vi "MBus Data Sort.vi"(3 "Error In":errorcluster, 4 "Raw Input Data":bool[](array[boolean]), 5 "Modbus master in":refnum<class "Modbus Master.lvclass">) -> (0 "Error Out":errorcluster, 1 "Cmd Value":bool[](array[boolean]), 2 "Modbus master out":refnum<class "Modbus Master.lvclass">)   [LabVIEW 2018]
uses:
  <vilib>/NI/Modbus Library/API/master/Modbus Master.lvclass
  CTL/FGV - R-W.ctl
panel:
  out "Supply 1 Voltage":u32
  out "Supply 2 Voltage":u32
  out "Remainder Data":bool[](array[boolean])
  out "Flash FB":bool[](array[boolean])
  out "Fault FB":bool[](array[boolean])
  out "Supply 2 Value":bool[](array[boolean])
  out "Supply 1 Value":bool[](array[boolean])
  out "System FB":bool[](array[boolean])
  out "Spares":bool[](array[boolean])
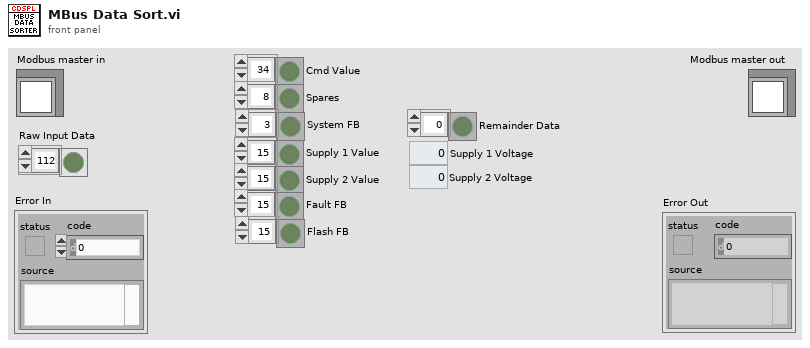
[diagram p1: front panel]
types:
  T1 = typedef "FGV - R-W.ctl" = enum16{"W", "R"}
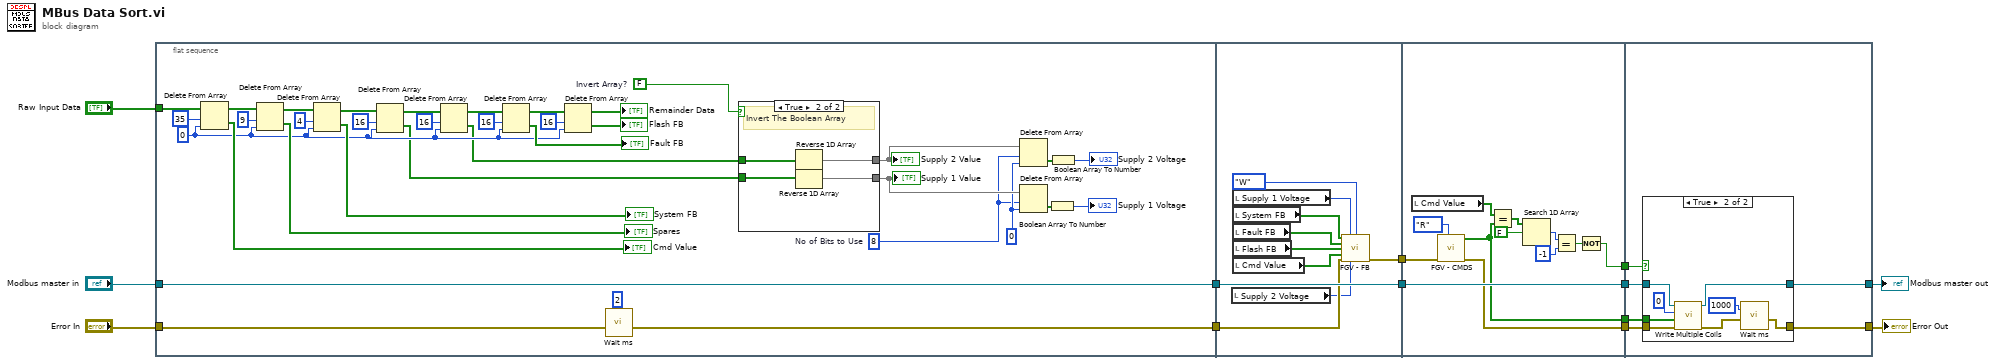
[diagram p0: block diagram]
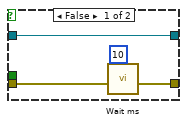
[diagram p3: hidden frame]
diagram:
  n1 = flat-sequence {
    tunnel: "Raw Input Data" -> [w49]
    tunnel: "Error In" -> [w16]
    tunnel: [w15] -> w10
    tunnel: "Modbus master in" -> [w14]
    tunnel: [w14] -> w8
    tunnel: w10 -> [w64]
    tunnel: w8 -> [w65]
    tunnel: [w63] -> w6
    tunnel: [w65] -> w5
    tunnel: w6 -> [w66]
    tunnel: w5 -> [w77]
    tunnel: [w75] -> w4
    tunnel: [w77] -> w3
    tunnel: [w68] -> w2
    tunnel: [w67] -> w1
    tunnel: [w80] -> w7
    tunnel: [w79] -> w11
    tunnel: w4 -> [w83]
    tunnel: w3 -> [w81]
    tunnel: w2 -> [w82]
    tunnel: w1 -> [w78]
    frame #0 {
      w22 = 8  # No of Bits to Use
      w23 = 0 ("index")
      w28 = FALSE  # Invert Array?
      w31 = 0 ("index")
      n2 = Delete From Array(array=w49, length=35, index=w31) -> (deleted portion=→"Cmd Value":bool[], array with subset deleted=w46:bool[])
      n3 = Delete From Array(array=w46, length=9, index=w31) -> (deleted portion=→"Spares":bool[], array with subset deleted=w43:bool[])
      n4 = Delete From Array(array=w43, length=4, index=w31) -> (deleted portion=→"System FB":bool[], array with subset deleted=w39:bool[])
      n5 = Delete From Array(array=w39, length=16, index=w31) -> (deleted portion=w26:bool[], array with subset deleted=w37:bool[])
      n6 = Delete From Array(array=w37, length=16, index=w31) -> (deleted portion=w27:bool[], array with subset deleted=w35:bool[])
      n7 = Delete From Array(array=w35, length=16, index=w31) -> (deleted portion=→"Fault FB":bool[], array with subset deleted=w33:bool[])
      n8 = Delete From Array(array=w33, length=16, index=w31) -> (deleted portion=→"Flash FB":bool[], array with subset deleted=→"Remainder Data":bool[])
      n9 = call "Wait ms.vi"("milliseconds to wait"=u32 2, "error in (no error)"=w16) -> ("error out"=w15:errorcluster)  [unwired: 9 in]
      n10 = case shown="True" w28 {
        tunnel: w27 -> [w51 w55]
        tunnel: [w51 w54] -> w25
        tunnel: w26 -> [w50 w53]
        tunnel: [w50 w52] -> w24
        frame False {
          # "Use Array as it is"
        }
        frame True {
          # "Invert The Boolean Array"
          n11 = Reverse 1D Array(array=w55) -> (reversed array=w54:bool[])
          n12 = Reverse 1D Array(array=w53) -> (reversed array=w52:bool[])
        }
      }
      "Supply 1 Value" <- w24
      "Supply 2 Value" <- w25
      n13 = Delete From Array(array=w25, length=w22, index=w23) -> (deleted portion=w21:bool[])  [unwired: 1 out]
      n14 = Delete From Array(array=w24, length=w22, index=w23) -> (deleted portion=w18:bool[])  [unwired: 1 out]
      n15 = Boolean Array To Number(Boolean array=w18) -> (number=→"Supply 1 Voltage":u32)
      n16 = Boolean Array To Number(Boolean array=w21) -> (number=→"Supply 2 Voltage":u32)
    }
    frame #1 {
      n17 = local read "Supply 2 Voltage"() -> (w61:u32)
      n18 = local read "Supply 1 Voltage"() -> (w60:u32)
      n19 = local read "System FB"() -> (w59:bool[])
      n20 = local read "Fault FB"() -> (w58:bool[])
      n21 = local read "Flash FB"() -> (w57:bool[])
      n22 = local read "Cmd Value"() -> (w56:bool[])
      n23 = call "FGV - FB.vi"("System FB"=w59, "Supply 1 Voltage"=w60, "Action"=FGV_-_R-W."W", "Fault FB"=w58, "Flash FB"=w57, "CMD FB"=w56, "error in (no error)"=w64, "Supply 2 Voltage"=w61) -> ("error out"=w63:errorcluster)  [unwired: 1 in, 6 out]
    }
    frame #2 {
      n24 = local read "Cmd Value"() -> (w69:bool[])
      n25 = call "FGV - CMDS.vi"("Action"=FGV_-_R-W."R", "error in (no error)"=w66) -> ("error out"=w75:errorcluster, "Cmd Out"=w68:bool[])  [unwired: 8 in]
      n26 = Equal?(x=w69, y=w68) -> (x = y?=w72:bool[])
      n27 = Search 1D Array(1D array=w72, element=FALSE) -> (index of element=w73:i32)  [unwired: 1 in]
      n28 = Equal?(x=w73, y=-1) -> (x = y?=w74:bool)
      n29 = Not(x=w74) -> (.not. x?=w67:bool)
    }
    frame #3 {
      n30 = case shown="True" w78 {
        tunnel: w81 -> [w87 w95]
        tunnel: w83 -> [w86 w94]
        tunnel: w82 -> [_ w92]
        tunnel: [w87 w91] -> w80
        tunnel: [w85 w88] -> w79
        frame False {
          n31 = call "Wait ms.vi"("milliseconds to wait"=u32 10, "error in (no error)"=w86) -> ("error out"=w85:errorcluster)  [unwired: 9 in]
        }
        frame True {
          n32 = call-dynamic "Write Multiple Coils.vi"("error in"=w94, "coils to write"=w92, "starting address"=u16 0, "Modbus master in"=w95) -> ("error out"=w89:errorcluster, "Modbus master out"=w91:refnum<class "Modbus Master.lvclass">)  [unwired: 6 in]
          n33 = call "Wait ms.vi"("milliseconds to wait"=u32 1000, "error in (no error)"=w89) -> ("error out"=w88:errorcluster)  [unwired: 9 in]
        }
      }
    }
  }
  "Error Out" <- w11
  "Modbus master out" <- w7
